vi "Convert_From_SI_Units.vi"(6 "Microsteps (MS=64)":dbl, 7 "Motor":u16(ring) items=["none", "1", "2", "3", "4", "all"], 8 "Output Unit":T1=enum."Meter", 10 "Input":dbl) -> (2 "Output":dbl)   [LabVIEW 2013]
uses:
  Unit_Control.ctl
  Constants.ctl
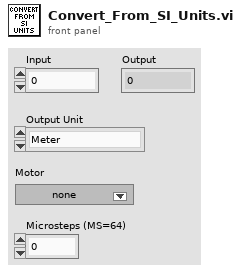
[diagram p1: front panel]
types:
  T1 = typedef "Unit_Control.ctl" = enum16{"Angle (Degrees)", "Rad", "Angle [TMC]", "Microsteps [TMC]", "Inches", "Nanometer", "Meter", "Centimeter", "Millimeter", "Micron", "Joule", "Electron Volts", "Hertz", "Terahertz", "Megahertz"}
  T2 = typedef "Constants.ctl" = dbl
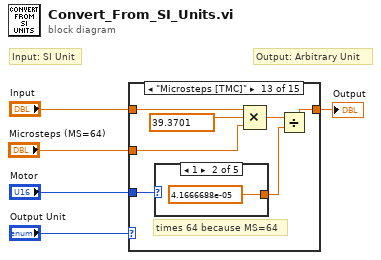
[diagram p0: block diagram]
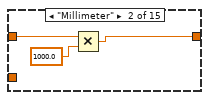
[diagram p3: hidden frame]
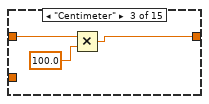
[diagram p4: hidden frame]
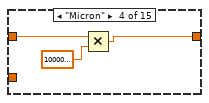
[diagram p5: hidden frame]
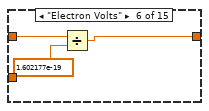
[diagram p7: hidden frame]
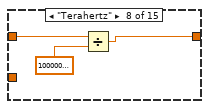
[diagram p9: hidden frame]
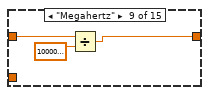
[diagram p10: hidden frame]
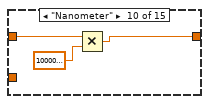
[diagram p11: hidden frame]
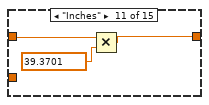
[diagram p12: hidden frame]
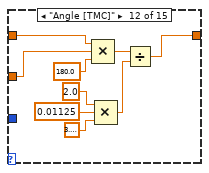
[diagram p13: hidden frame]
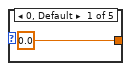
[diagram p14: hidden frame]
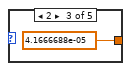
[diagram p15: hidden frame]
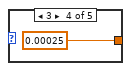
[diagram p16: hidden frame]
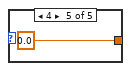
[diagram p17: hidden frame]
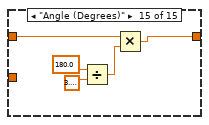
[diagram p19: hidden frame]
diagram:
  # "Output: Arbitrary Unit"
  # "Input: SI Unit"
  n1 = case shown="\"Microsteps [TMC]\"" "Output Unit" {
    tunnel: "Input" -> [w6 w9 w12 w15 w16 w19 w20 w23 w26 w29 w31 w41 w46 w54 w57]
    tunnel: [w6 w8 w10 w14 w16 w18 w20 w22 w25 w28 w30 w37 w45 w54 w55] -> w5
    tunnel: "Motor" -> [_ _ _ _ _ _ _ _ _ _ _ _ w44 _ _]
    tunnel: "Microsteps (MS=64)" -> [_ _ _ _ _ _ _ _ _ _ _ w33 w43 _ _]
    frame "Meter", Default {
    }
    frame "Millimeter" {
      n2 = Multiply(x=w9, y=1000.0) -> (x*y=w8:dbl)
    }
    frame "Centimeter" {
      n3 = Multiply(x=w12, y=100.0) -> (x*y=w10:dbl)
    }
    frame "Micron" {
      n4 = Multiply(x=w15, y=1000000.0) -> (x*y=w14:dbl)
    }
    frame "Joule" {
    }
    frame "Electron Volts" {
      w17 = T2 1.602177e-19 items=["pi (Number)"=3.141593, "e [As]"=1.602177e-19, "h [Js]"=6.62607e-34, "c [m/s]"=299792500.0, "e (Number)"=2.718282] ("Constants")
      n5 = Divide(x=w19, y=w17) -> (x/y=w18:T2)
    }
    frame "Hertz" {
    }
    frame "Terahertz" {
      n6 = Divide(x=w23, y=1000000000000.0) -> (x/y=w22:dbl)
    }
    frame "Megahertz" {
      n7 = Divide(x=w26, y=1000000.0) -> (x/y=w25:dbl)
    }
    frame "Nanometer" {
      n8 = Multiply(x=w29, y=1000000000.0) -> (x*y=w28:dbl)
    }
    frame "Inches" {
      n9 = Multiply(x=w31, y=39.3701) -> (x*y=w30:dbl)
    }
    frame "Angle [TMC]" {
      n10 = Compound Arithmetic op=MULTIPLY(w41, w33, 180.0 ("y")) -> (w39:dbl)
      n11 = Compound Arithmetic op=MULTIPLY(2.0 ("x"), 0.01125, 3.141592653589793) -> (w38:dbl)
      n12 = Divide(x=w39, y=w38) -> (x/y=w37:dbl)
    }
    frame "Microsteps [TMC]" {
      # "times 64 because MS=64"
      n13 = case shown="1" w44 {
        tunnel: [0.0 4.1666688e-05 4.1666688e-05 0.00025 0.0] -> w42
        frame 0, Default {
        }
        frame 1 {
        }
        frame 2 {
        }
        frame 3 {
        }
        frame 4 {
        }
      }
      n14 = Compound Arithmetic op=MULTIPLY(w46, 39.3701, w43) -> (w47:dbl)
      n15 = Divide(x=w47, y=w42) -> (x/y=w45:dbl)
    }
    frame "Rad" {
    }
    frame "Angle (Degrees)" {
      n16 = Divide(x=180.0 ("y"), y=3.141592653589793) -> (x/y=w56:dbl)
      n17 = Multiply(x=w57, y=w56) -> (x*y=w55:dbl)
    }
  }
  "Output" <- w5
